vi "conversion_Conf_FPGA_graphXY.vi"(11 "Config FPGA":T1 {"t_periode" min=1 max=999999 step=1}) -> (3 "appended array":cluster{cluster{"t_periode":i32, dbl}[]}[](array[cluster]))   [LabVIEW 2023]
uses:
  configFPGA.ctl
  tempsI32.ctl
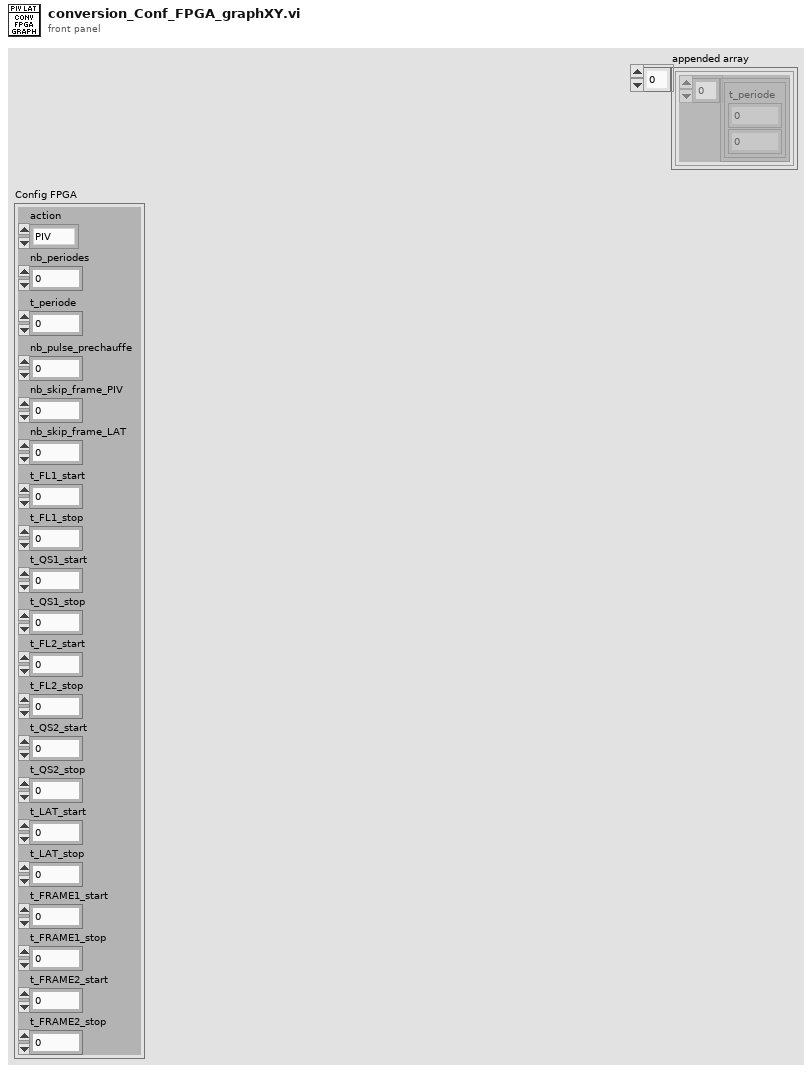
[diagram p1: front panel]
types:
  T1 = typedef "configFPGA.ctl" = cluster{"action":enum8{"PIV", "PIV + LAT", "LAT", "STOP"}, "nb_periodes":u16, "t_periode":u32, "nb_pulse_prechauffe":u8, "nb_skip_frame_PIV":u8, "nb_skip_frame_LAT":u8, "t_FL1_start":u32, "t_FL1_stop":u32, "t_QS1_start":u32, "t_QS1_stop":u32, "t_FL2_start":u32, "t_FL2_stop":u32, "t_QS2_start":u32, "t_QS2_stop":u32, "t_LAT_start":u32, "t_LAT_stop":u32, "t_FRAME1_start":u32, "t_FRAME1_stop":u32, "t_FRAME2_start":u32, "t_FRAME2_stop":u32}
  T2 = typedef "tempsI32.ctl" = cluster{"t_periode":i32, "t_FL1_start":i32, "t_FL1_stop":i32, "t_QS1_start":i32, "t_QS1_stop":i32, "t_FL2_start":i32, "t_FL2_stop":i32, "t_QS2_start":i32, "t_QS2_stop":i32, "t_LAT_start":i32, "t_LAT_stop":i32, "t_FRAME1_start":i32, "t_FRAME1_stop":i32, "t_FRAME2_start":i32, "t_FRAME2_stop":i32}
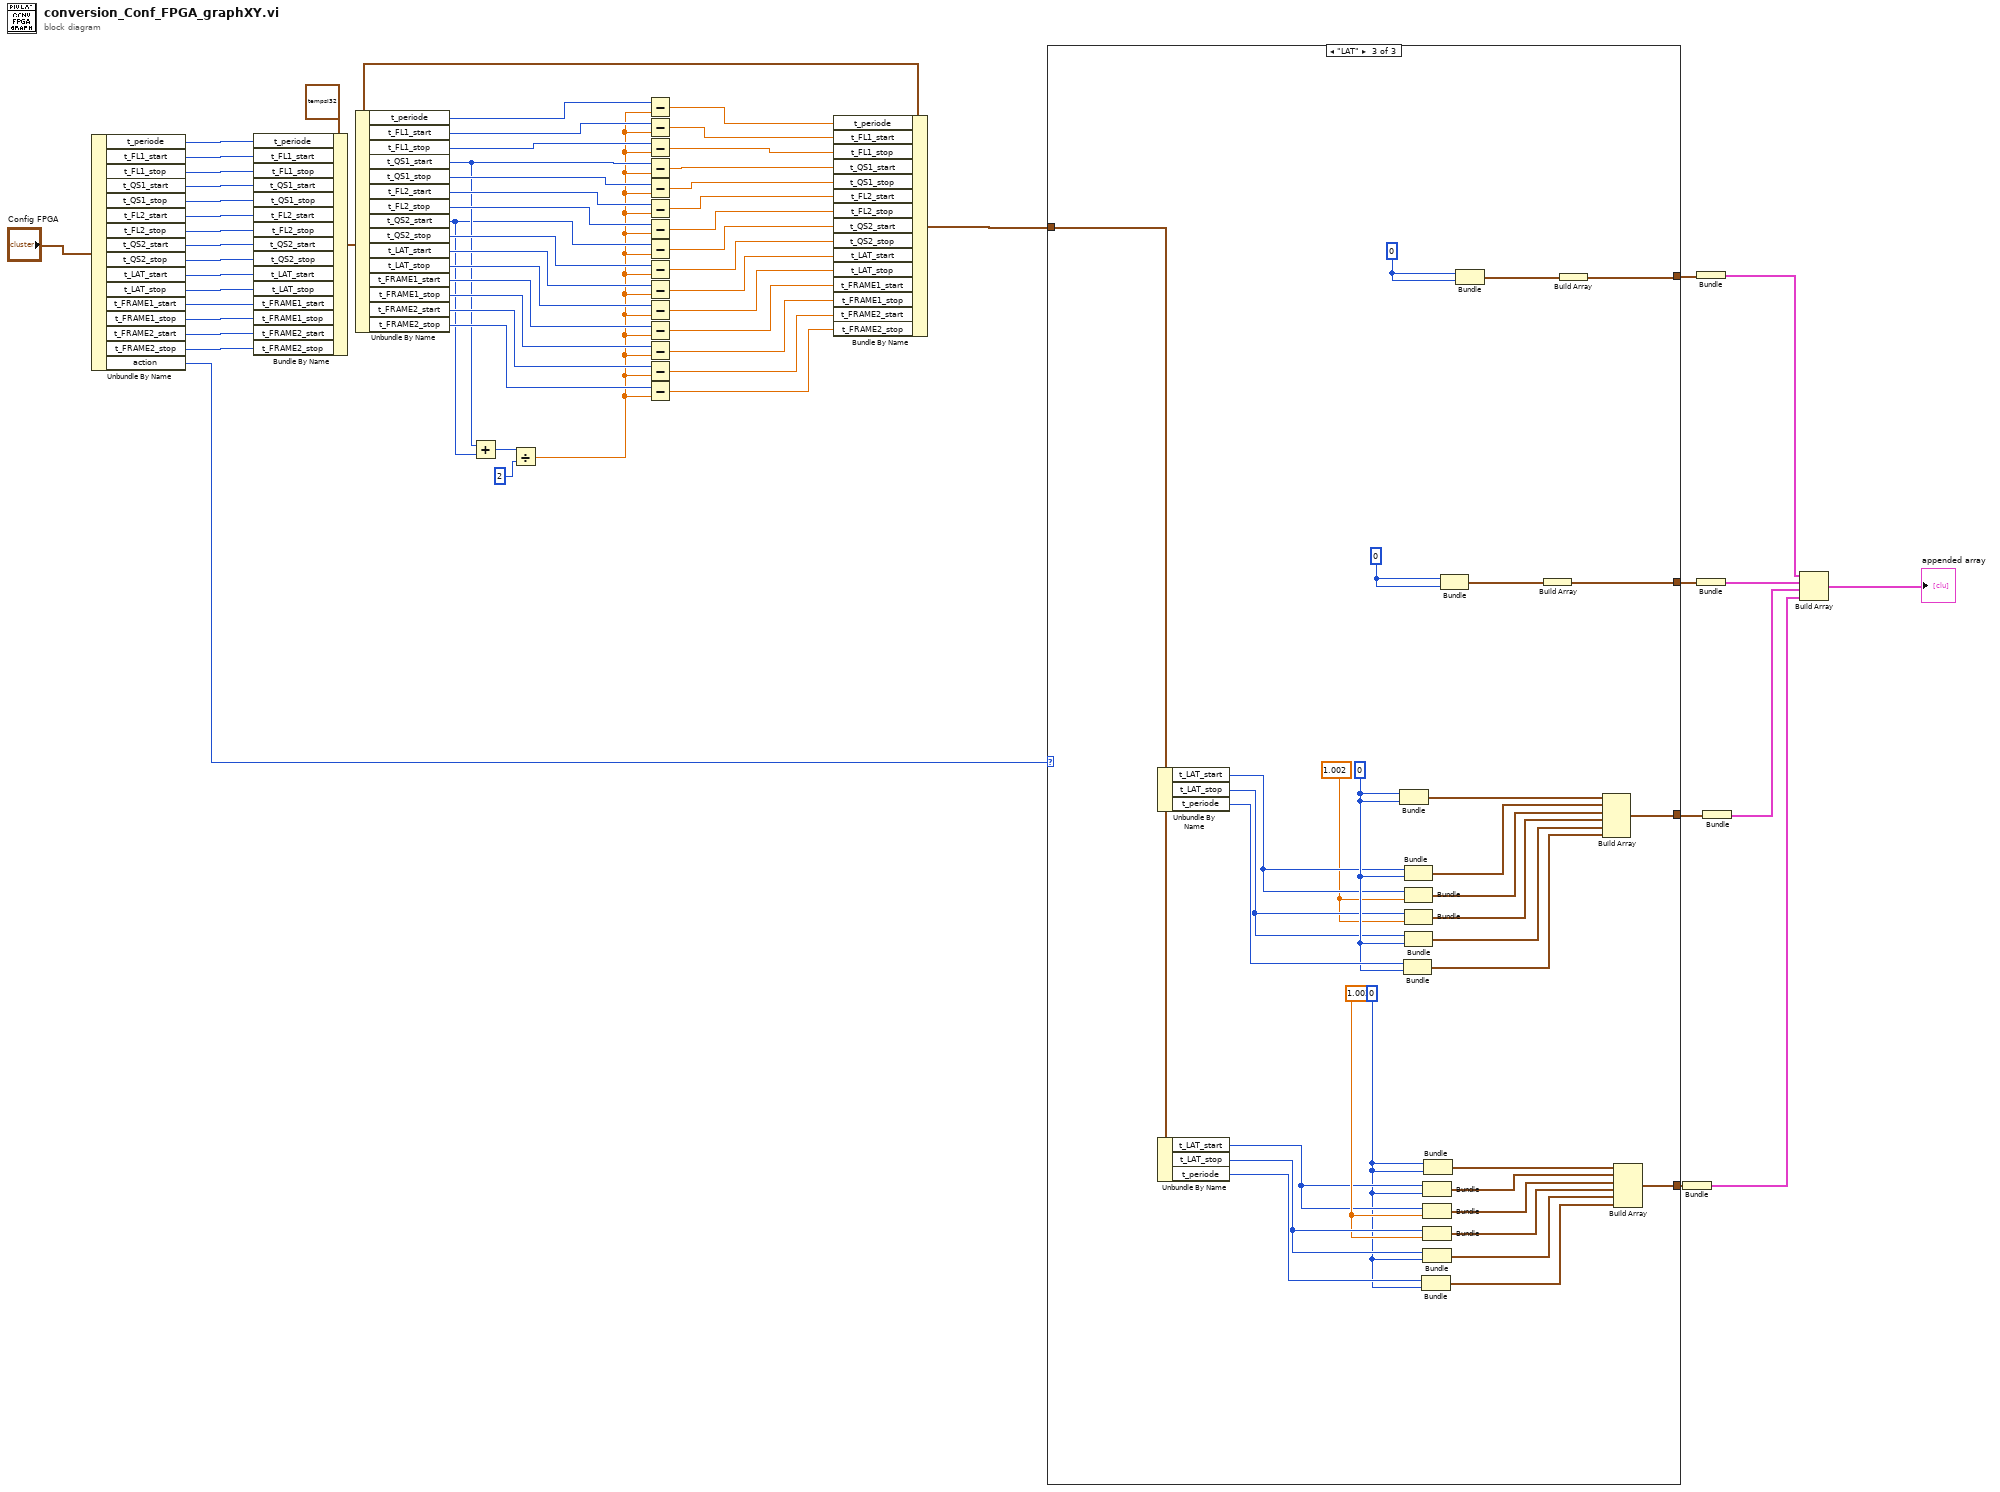
[diagram p0: block diagram]
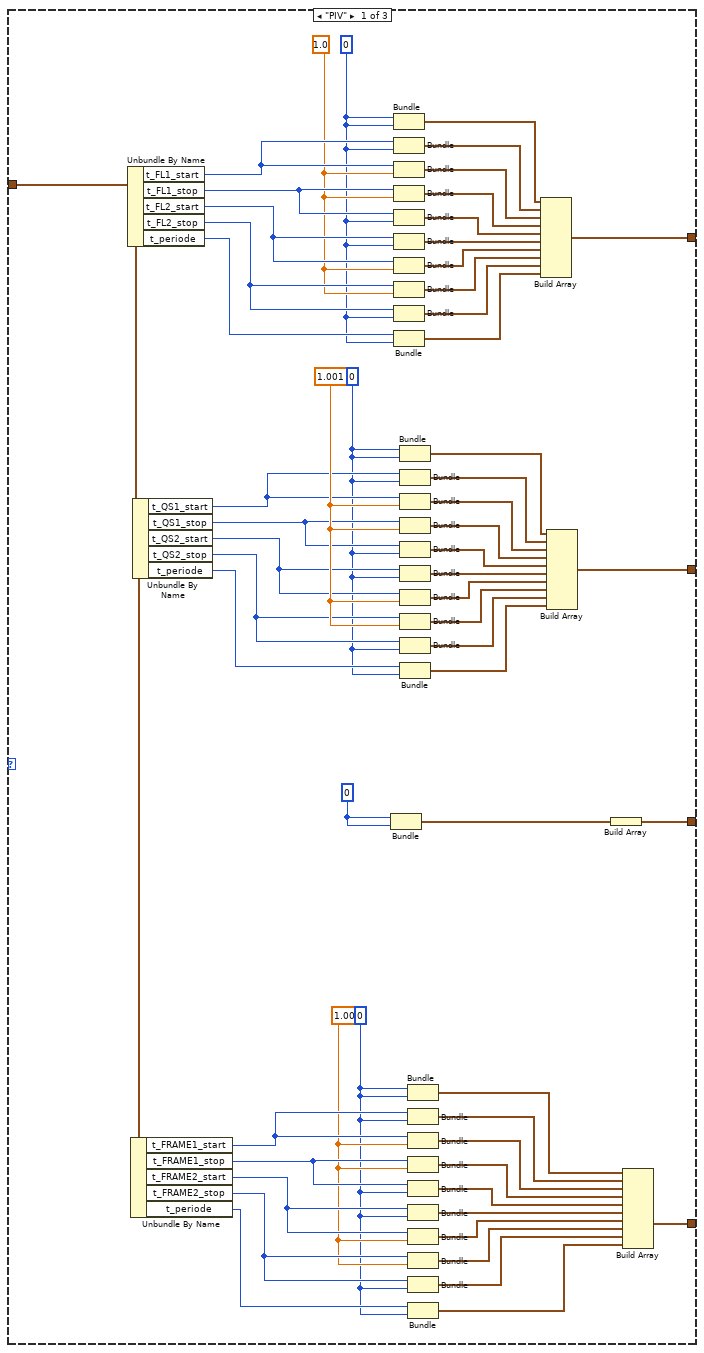
[diagram p2: hidden frame]
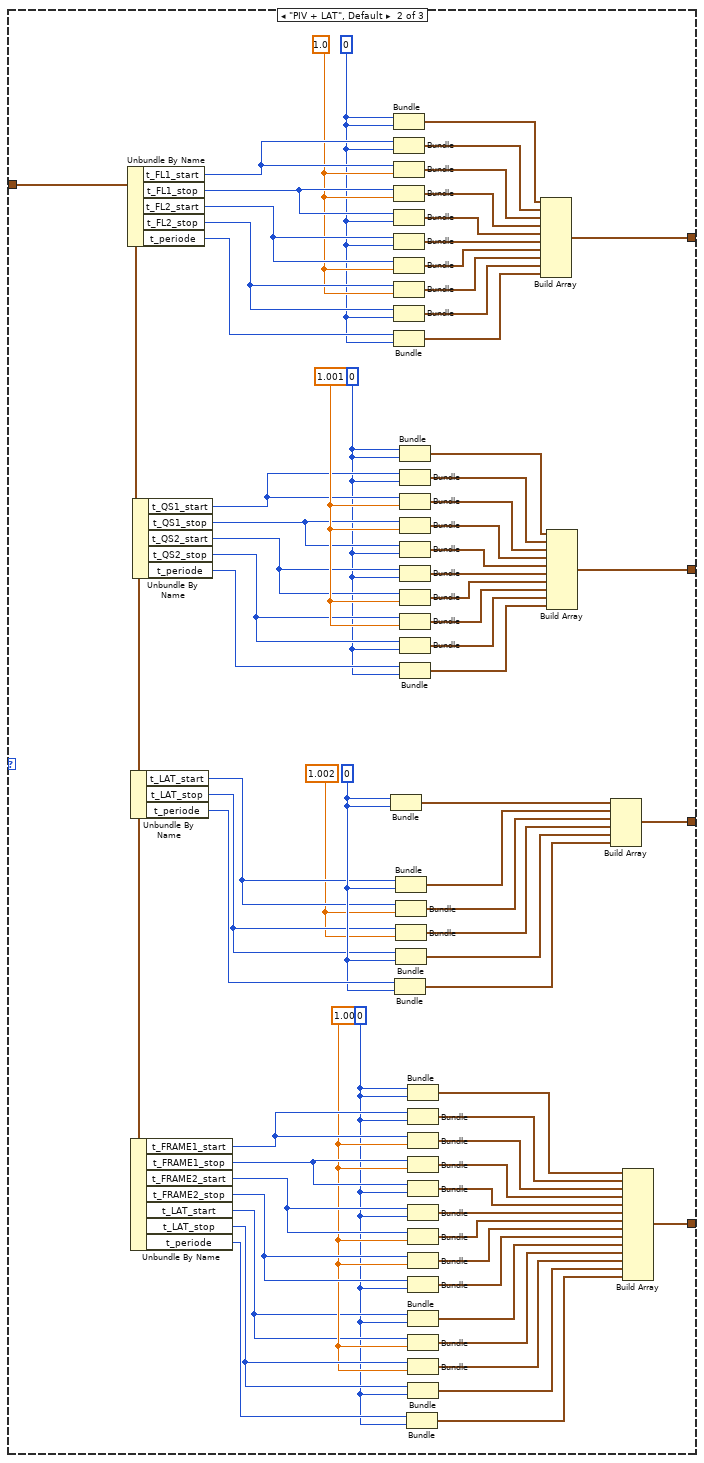
[diagram p3: hidden frame]
diagram:
  n1 = Unbundle By Name("Config FPGA") -> ("t_periode"=w24:u32, "t_FL1_start"=w23:u32, "t_FL1_stop"=w22:u32, "t_QS1_start"=w21:u32, "t_QS1_stop"=w20:u32, "t_FL2_start"=w19:u32, "t_FL2_stop"=w18:u32, "t_QS2_start"=w17:u32, "t_QS2_stop"=w16:u32, "t_LAT_start"=w15:u32, "t_LAT_stop"=w14:u32, "t_FRAME1_start"=w10:u32, "t_FRAME1_stop"=w11:u32, "t_FRAME2_start"=w12:u32, "t_FRAME2_stop"=w13:u32, "action"=w1:enum8{"PIV", "PIV + LAT", "LAT", "STOP"})
  n2 = Bundle By Name(cluster=T2 {"t_periode"=1000000, "t_FL1_start"=0, "t_FL1_stop"=10, "t_QS1_start"=180, "t_QS1_stop"=190, "t_FL2_start"=10000, "t_FL2_stop"=10010, "t_QS2_start"=10180, "t_QS2_stop"=10190, "t_LAT_start"=17180, "t_LAT_stop"=22180, "t_FRAME1_start"=170, "t_FRAME1_stop"=190, "t_FRAME2_start"=10170, "t_FRAME2_stop"=10190} ("Config FPGA"), "t_periode"=w24, "t_FL1_start"=w23, "t_FL1_stop"=w22, "t_QS1_start"=w21, "t_QS1_stop"=w20, "t_FL2_start"=w19, "t_FL2_stop"=w18, "t_QS2_start"=w17, "t_QS2_stop"=w16, "t_LAT_start"=w15, "t_LAT_stop"=w14, "t_FRAME1_start"=w10, "t_FRAME1_stop"=w11, "t_FRAME2_start"=w12, "t_FRAME2_stop"=w13) -> (w26:T2)
  n3 = Unbundle By Name(w26) -> ("t_periode"=w58:i32, "t_FL1_start"=w57:i32, "t_FL1_stop"=w56:i32, "t_QS1_start"=w9:i32, "t_QS1_stop"=w55:i32, "t_FL2_start"=w54:i32, "t_FL2_stop"=w30:i32, "t_QS2_start"=w8:i32, "t_QS2_stop"=w53:i32, "t_LAT_start"=w52:i32, "t_LAT_stop"=w29:i32, "t_FRAME1_start"=w51:i32, "t_FRAME1_stop"=w50:i32, "t_FRAME2_start"=w49:i32, "t_FRAME2_stop"=w48:i32)
  n4 = Add(x=w9, y=w8) -> (x+y=w31:i32)
  n5 = Divide(x=w31, y=u32 2) -> (x/y=w7:dbl)
  n6 = Subtract(x=w58, y=w7) -> (x-y=w47:dbl)
  n7 = Subtract(x=w57, y=w7) -> (x-y=w46:dbl)
  n8 = Subtract(x=w56, y=w7) -> (x-y=w45:dbl)
  n9 = Subtract(x=w9, y=w7) -> (x-y=w44:dbl)
  n10 = Subtract(x=w55, y=w7) -> (x-y=w43:dbl)
  n11 = Subtract(x=w54, y=w7) -> (x-y=w42:dbl)
  n12 = Subtract(x=w30, y=w7) -> (x-y=w41:dbl)
  n13 = Subtract(x=w8, y=w7) -> (x-y=w40:dbl)
  n14 = Subtract(x=w53, y=w7) -> (x-y=w39:dbl)
  n15 = Subtract(x=w52, y=w7) -> (x-y=w38:dbl)
  n16 = Subtract(x=w29, y=w7) -> (x-y=w37:dbl)
  n17 = Subtract(x=w51, y=w7) -> (x-y=w36:dbl)
  n18 = Subtract(x=w50, y=w7) -> (x-y=w35:dbl)
  n19 = Subtract(x=w49, y=w7) -> (x-y=w34:dbl)
  n20 = Subtract(x=w48, y=w7) -> (x-y=w33:dbl)
  n21 = Bundle By Name(cluster=w26, "t_periode"=w47, "t_FL1_start"=w46, "t_FL1_stop"=w45, "t_QS1_start"=w44, "t_QS1_stop"=w43, "t_FL2_start"=w42, "t_FL2_stop"=w41, "t_QS2_start"=w40, "t_QS2_stop"=w39, "t_LAT_start"=w38, "t_LAT_stop"=w37, "t_FRAME1_start"=w36, "t_FRAME1_stop"=w35, "t_FRAME2_start"=w34, "t_FRAME2_stop"=w33) -> (w32:T2)
  n22 = case shown="\"LAT\"" w1 {
    tunnel: [w88 w161 w223] -> w62
    tunnel: [w87 w160 w222] -> w61
    tunnel: w32 -> [w84 w157 w220]
    tunnel: [w83 w156 w219] -> w5
    tunnel: [w82 w155 w195] -> w3
    frame "PIV" {
      w67 = 0
      w64 = 0
      w65 = 1.003
      w85 = 0
      w93 = 1.001
      w86 = 0
      w116 = 1.0
      n23 = Unbundle By Name(w84) -> ("t_FL1_start"=w120:i32, "t_FL1_stop"=w119:i32, "t_FL2_start"=w118:i32, "t_FL2_stop"=w117:i32, "t_periode"=w115:i32)
      n24 = Unbundle By Name(w84) -> ("t_FRAME1_start"=w81:i32, "t_FRAME1_stop"=w80:i32, "t_FRAME2_start"=w79:i32, "t_FRAME2_stop"=w78:i32, "t_periode"=w68:i32)
      n25 = Unbundle By Name(w84) -> ("t_QS1_start"=w89:i32, "t_QS1_stop"=w90:i32, "t_QS2_start"=w91:i32, "t_QS2_stop"=w92:i32, "t_periode"=w94:i32)
      n26 = Bundle(w67, w67) -> (w66:cluster{i32, i32})  [unwired: 1 in]
      n27 = Bundle(w86, w86) -> (w114:cluster{i32, i32})  [unwired: 1 in]
      n28 = Bundle("t_FL1_start"=w120, w86) -> (w113:cluster{"t_FL1_start":i32, i32})  [unwired: 1 in]
      n29 = Bundle("t_FL1_start"=w120, w116) -> (w112:cluster{"t_FL1_start":i32, dbl})  [unwired: 1 in]
      n30 = Bundle("t_FL1_stop"=w119, w116) -> (w111:cluster{"t_FL1_stop":i32, dbl})  [unwired: 1 in]
      n31 = Bundle("t_FL1_stop"=w119, w86) -> (w110:cluster{"t_FL1_stop":i32, i32})  [unwired: 1 in]
      n32 = Bundle("t_FL2_start"=w118, w86) -> (w109:cluster{"t_FL2_start":i32, i32})  [unwired: 1 in]
      n33 = Bundle("t_FL2_start"=w118, w116) -> (w108:cluster{"t_FL2_start":i32, dbl})  [unwired: 1 in]
      n34 = Bundle("t_FL2_stop"=w117, w116) -> (w107:cluster{"t_FL2_stop":i32, dbl})  [unwired: 1 in]
      n35 = Bundle("t_FL2_stop"=w117, w86) -> (w106:cluster{"t_FL2_stop":i32, i32})  [unwired: 1 in]
      n36 = Bundle("t_periode"=w115, w86) -> (w105:cluster{"t_periode":i32, i32})  [unwired: 1 in]
      n37 = Bundle(w85, w85) -> (w95:cluster{i32, i32})  [unwired: 1 in]
      n38 = Bundle("t_QS1_start"=w89, w85) -> (w96:cluster{"t_QS1_start":i32, i32})  [unwired: 1 in]
      n39 = Bundle("t_QS1_start"=w89, w93) -> (w97:cluster{"t_QS1_start":i32, dbl})  [unwired: 1 in]
      n40 = Bundle("t_QS1_stop"=w90, w93) -> (w98:cluster{"t_QS1_stop":i32, dbl})  [unwired: 1 in]
      n41 = Bundle("t_QS1_stop"=w90, w85) -> (w99:cluster{"t_QS1_stop":i32, i32})  [unwired: 1 in]
      n42 = Bundle("t_QS2_start"=w91, w85) -> (w100:cluster{"t_QS2_start":i32, i32})  [unwired: 1 in]
      n43 = Bundle("t_QS2_start"=w91, w93) -> (w101:cluster{"t_QS2_start":i32, dbl})  [unwired: 1 in]
      n44 = Bundle("t_QS2_stop"=w92, w93) -> (w102:cluster{"t_QS2_stop":i32, dbl})  [unwired: 1 in]
      n45 = Bundle("t_QS2_stop"=w92, w85) -> (w103:cluster{"t_QS2_stop":i32, i32})  [unwired: 1 in]
      n46 = Bundle("t_periode"=w94, w85) -> (w104:cluster{"t_periode":i32, i32})  [unwired: 1 in]
      n47 = Bundle(w64, w64) -> (w77:cluster{i32, i32})  [unwired: 1 in]
      n48 = Bundle("t_FRAME1_start"=w81, w64) -> (w76:cluster{"t_FRAME1_start":i32, i32})  [unwired: 1 in]
      n49 = Bundle("t_FRAME1_start"=w81, w65) -> (w75:cluster{"t_FRAME1_start":i32, dbl})  [unwired: 1 in]
      n50 = Bundle("t_FRAME1_stop"=w80, w65) -> (w74:cluster{"t_FRAME1_stop":i32, dbl})  [unwired: 1 in]
      n51 = Bundle("t_FRAME1_stop"=w80, w64) -> (w73:cluster{"t_FRAME1_stop":i32, i32})  [unwired: 1 in]
      n52 = Bundle("t_FRAME2_start"=w79, w64) -> (w72:cluster{"t_FRAME2_start":i32, i32})  [unwired: 1 in]
      n53 = Bundle("t_FRAME2_start"=w79, w65) -> (w71:cluster{"t_FRAME2_start":i32, dbl})  [unwired: 1 in]
      n54 = Bundle("t_FRAME2_stop"=w78, w65) -> (w70:cluster{"t_FRAME2_stop":i32, dbl})  [unwired: 1 in]
      n55 = Bundle("t_FRAME2_stop"=w78, w64) -> (w69:cluster{"t_FRAME2_stop":i32, i32})  [unwired: 1 in]
      n56 = Bundle("t_periode"=w68, w64) -> (w63:cluster{"t_periode":i32, i32})  [unwired: 1 in]
      n57 = Build Array(w114, w113, w112, w111, w110, w109, w108, w107, w106, w105) -> (w82:cluster{"t_periode":i32, dbl}[])
      n58 = Build Array(w95, w96, w97, w98, w99, w100, w101, w102, w103, w104) -> (w83:cluster{"t_periode":i32, dbl}[])
      n59 = Build Array(w66) -> (w87:cluster{i32, i32}[])
      n60 = Build Array(w77, w76, w75, w74, w73, w72, w71, w70, w69, w63) -> (w88:cluster{"t_periode":i32, dbl}[])
    }
    frame "PIV + LAT", Default {
      w128 = 0
      w124 = 1.002
      w121 = 0
      w123 = 1.003
      w158 = 0
      w166 = 1.001
      w159 = 0
      w189 = 1.0
      n61 = Unbundle By Name(w157) -> ("t_FL1_start"=w193:i32, "t_FL1_stop"=w192:i32, "t_FL2_start"=w191:i32, "t_FL2_stop"=w190:i32, "t_periode"=w188:i32)
      n62 = Unbundle By Name(w157) -> ("t_LAT_start"=w125:i32, "t_LAT_stop"=w127:i32, "t_periode"=w129:i32)
      n63 = Unbundle By Name(w157) -> ("t_FRAME1_start"=w154:i32, "t_FRAME1_stop"=w153:i32, "t_FRAME2_start"=w152:i32, "t_FRAME2_stop"=w151:i32, "t_LAT_start"=w122:i32, "t_LAT_stop"=w141:i32, "t_periode"=w140:i32)
      n64 = Unbundle By Name(w157) -> ("t_QS1_start"=w162:i32, "t_QS1_stop"=w163:i32, "t_QS2_start"=w164:i32, "t_QS2_stop"=w165:i32, "t_periode"=w167:i32)
      n65 = Bundle(w128, w128) -> (w126:cluster{i32, i32})  [unwired: 1 in]
      n66 = Bundle(w159, w159) -> (w187:cluster{i32, i32})  [unwired: 1 in]
      n67 = Bundle("t_FL1_start"=w193, w159) -> (w186:cluster{"t_FL1_start":i32, i32})  [unwired: 1 in]
      n68 = Bundle("t_FL1_start"=w193, w189) -> (w185:cluster{"t_FL1_start":i32, dbl})  [unwired: 1 in]
      n69 = Bundle("t_FL1_stop"=w192, w189) -> (w184:cluster{"t_FL1_stop":i32, dbl})  [unwired: 1 in]
      n70 = Bundle("t_FL1_stop"=w192, w159) -> (w183:cluster{"t_FL1_stop":i32, i32})  [unwired: 1 in]
      n71 = Bundle("t_FL2_start"=w191, w159) -> (w182:cluster{"t_FL2_start":i32, i32})  [unwired: 1 in]
      n72 = Bundle("t_FL2_start"=w191, w189) -> (w181:cluster{"t_FL2_start":i32, dbl})  [unwired: 1 in]
      n73 = Bundle("t_FL2_stop"=w190, w189) -> (w180:cluster{"t_FL2_stop":i32, dbl})  [unwired: 1 in]
      n74 = Bundle("t_FL2_stop"=w190, w159) -> (w179:cluster{"t_FL2_stop":i32, i32})  [unwired: 1 in]
      n75 = Bundle("t_periode"=w188, w159) -> (w178:cluster{"t_periode":i32, i32})  [unwired: 1 in]
      n76 = Bundle("t_periode"=w129, w128) -> (w134:cluster{"t_periode":i32, i32})  [unwired: 1 in]
      n77 = Bundle("t_LAT_start"=w125, w128) -> (w130:cluster{"t_LAT_start":i32, i32})  [unwired: 1 in]
      n78 = Bundle("t_LAT_start"=w125, w124) -> (w131:cluster{"t_LAT_start":i32, dbl})  [unwired: 1 in]
      n79 = Bundle("t_LAT_stop"=w127, w124) -> (w132:cluster{"t_LAT_stop":i32, dbl})  [unwired: 1 in]
      n80 = Bundle("t_LAT_stop"=w127, w128) -> (w133:cluster{"t_LAT_stop":i32, i32})  [unwired: 1 in]
      n81 = Bundle(w158, w158) -> (w168:cluster{i32, i32})  [unwired: 1 in]
      n82 = Bundle("t_QS1_start"=w162, w158) -> (w169:cluster{"t_QS1_start":i32, i32})  [unwired: 1 in]
      n83 = Bundle("t_QS1_start"=w162, w166) -> (w170:cluster{"t_QS1_start":i32, dbl})  [unwired: 1 in]
      n84 = Bundle("t_QS1_stop"=w163, w166) -> (w171:cluster{"t_QS1_stop":i32, dbl})  [unwired: 1 in]
      n85 = Bundle("t_QS1_stop"=w163, w158) -> (w172:cluster{"t_QS1_stop":i32, i32})  [unwired: 1 in]
      n86 = Bundle("t_QS2_start"=w164, w158) -> (w173:cluster{"t_QS2_start":i32, i32})  [unwired: 1 in]
      n87 = Bundle("t_QS2_start"=w164, w166) -> (w174:cluster{"t_QS2_start":i32, dbl})  [unwired: 1 in]
      n88 = Bundle("t_QS2_stop"=w165, w166) -> (w175:cluster{"t_QS2_stop":i32, dbl})  [unwired: 1 in]
      n89 = Bundle("t_QS2_stop"=w165, w158) -> (w176:cluster{"t_QS2_stop":i32, i32})  [unwired: 1 in]
      n90 = Bundle("t_periode"=w167, w158) -> (w177:cluster{"t_periode":i32, i32})  [unwired: 1 in]
      n91 = Bundle("t_periode"=w140, w121) -> (w135:cluster{"t_periode":i32, i32})  [unwired: 1 in]
      n92 = Bundle(w121, w121) -> (w150:cluster{i32, i32})  [unwired: 1 in]
      n93 = Bundle("t_FRAME1_start"=w154, w121) -> (w149:cluster{"t_FRAME1_start":i32, i32})  [unwired: 1 in]
      n94 = Bundle("t_FRAME1_start"=w154, w123) -> (w148:cluster{"t_FRAME1_start":i32, dbl})  [unwired: 1 in]
      n95 = Bundle("t_FRAME1_stop"=w153, w123) -> (w147:cluster{"t_FRAME1_stop":i32, dbl})  [unwired: 1 in]
      n96 = Bundle("t_FRAME1_stop"=w153, w121) -> (w146:cluster{"t_FRAME1_stop":i32, i32})  [unwired: 1 in]
      n97 = Bundle("t_FRAME2_start"=w152, w121) -> (w145:cluster{"t_FRAME2_start":i32, i32})  [unwired: 1 in]
      n98 = Bundle("t_FRAME2_start"=w152, w123) -> (w144:cluster{"t_FRAME2_start":i32, dbl})  [unwired: 1 in]
      n99 = Bundle("t_FRAME2_stop"=w151, w123) -> (w143:cluster{"t_FRAME2_stop":i32, dbl})  [unwired: 1 in]
      n100 = Bundle("t_FRAME2_stop"=w151, w121) -> (w142:cluster{"t_FRAME2_stop":i32, i32})  [unwired: 1 in]
      n101 = Bundle("t_LAT_start"=w122, w121) -> (w139:cluster{"t_LAT_start":i32, i32})  [unwired: 1 in]
      n102 = Bundle("t_LAT_start"=w122, w123) -> (w138:cluster{"t_LAT_start":i32, dbl})  [unwired: 1 in]
      n103 = Bundle("t_LAT_stop"=w141, w123) -> (w137:cluster{"t_LAT_stop":i32, dbl})  [unwired: 1 in]
      n104 = Bundle("t_LAT_stop"=w141, w121) -> (w136:cluster{"t_LAT_stop":i32, i32})  [unwired: 1 in]
      n105 = Build Array(w187, w186, w185, w184, w183, w182, w181, w180, w179, w178) -> (w155:cluster{"t_periode":i32, dbl}[])
      n106 = Build Array(w168, w169, w170, w171, w172, w173, w174, w175, w176, w177) -> (w156:cluster{"t_periode":i32, dbl}[])
      n107 = Build Array(w126, w130, w131, w132, w133, w134) -> (w160:cluster{"t_periode":i32, dbl}[])
      n108 = Build Array(w150, w149, w148, w147, w146, w145, w144, w143, w142, w139, w138, w137, w136, w135) -> (w161:cluster{"t_periode":i32, dbl}[])
    }
    frame "LAT" {
      w196 = 0
      w205 = 0
      w201 = 1.002
      w198 = 0
      w200 = 1.003
      w221 = 0
      n109 = Unbundle By Name(w220) -> ("t_LAT_start"=w202:i32, "t_LAT_stop"=w204:i32, "t_periode"=w206:i32)
      n110 = Unbundle By Name(w220) -> ("t_LAT_start"=w199:i32, "t_LAT_stop"=w218:i32, "t_periode"=w217:i32)
      n111 = Bundle(w205, w205) -> (w203:cluster{i32, i32})  [unwired: 1 in]
      n112 = Bundle("t_periode"=w206, w205) -> (w211:cluster{"t_periode":i32, i32})  [unwired: 1 in]
      n113 = Bundle("t_LAT_start"=w202, w205) -> (w207:cluster{"t_LAT_start":i32, i32})  [unwired: 1 in]
      n114 = Bundle("t_LAT_start"=w202, w201) -> (w208:cluster{"t_LAT_start":i32, dbl})  [unwired: 1 in]
      n115 = Bundle("t_LAT_stop"=w204, w201) -> (w209:cluster{"t_LAT_stop":i32, dbl})  [unwired: 1 in]
      n116 = Bundle("t_LAT_stop"=w204, w205) -> (w210:cluster{"t_LAT_stop":i32, i32})  [unwired: 1 in]
      n117 = Bundle("t_periode"=w217, w198) -> (w212:cluster{"t_periode":i32, i32})  [unwired: 1 in]
      n118 = Bundle("t_LAT_start"=w199, w198) -> (w216:cluster{"t_LAT_start":i32, i32})  [unwired: 1 in]
      n119 = Bundle("t_LAT_start"=w199, w200) -> (w215:cluster{"t_LAT_start":i32, dbl})  [unwired: 1 in]
      n120 = Bundle("t_LAT_stop"=w218, w200) -> (w214:cluster{"t_LAT_stop":i32, dbl})  [unwired: 1 in]
      n121 = Bundle("t_LAT_stop"=w218, w198) -> (w213:cluster{"t_LAT_stop":i32, i32})  [unwired: 1 in]
      n122 = Bundle(w198, w198) -> (w194:cluster{i32, i32})  [unwired: 1 in]
      n123 = Bundle(w221, w221) -> (w224:cluster{i32, i32})  [unwired: 1 in]
      n124 = Bundle(w196, w196) -> (w197:cluster{i32, i32})  [unwired: 1 in]
      n125 = Build Array(w224) -> (w219:cluster{i32, i32}[])
      n126 = Build Array(w197) -> (w195:cluster{i32, i32}[])
      n127 = Build Array(w203, w207, w208, w209, w210, w211) -> (w222:cluster{"t_periode":i32, dbl}[])
      n128 = Build Array(w194, w216, w215, w214, w213, w212) -> (w223:cluster{"t_periode":i32, dbl}[])
    }
  }
  n129 = Bundle(w62) -> (w59:cluster{cluster{"t_periode":i32, dbl}[]})  [unwired: 1 in]
  n130 = Bundle(w3) -> (w2:cluster{cluster{"t_periode":i32, dbl}[]})  [unwired: 1 in]
  n131 = Bundle(w5) -> (w4:cluster{cluster{"t_periode":i32, dbl}[]})  [unwired: 1 in]
  n132 = Bundle(w61) -> (w60:cluster{cluster{"t_periode":i32, dbl}[]})  [unwired: 1 in]
  n133 = Build Array(w2, w4, w60, w59) -> (→"appended array":cluster{cluster{"t_periode":i32, dbl}[]}[])
